vi "Write to Active Buffer.vi"(8 "error in (no error)":errorcluster, 10 "Data":string, 11 "Terminal in":refnum<class "Terminal.lvclass">) -> (0 "error out":errorcluster, 3 "Terminal out":refnum<class "Terminal.lvclass">)   [LabVIEW 2020, in "Terminal.lvlib" / "Terminal.lvclass"]
uses:
  Terminal.lvclass
  Terminal.lvclass/Terminal.ctl
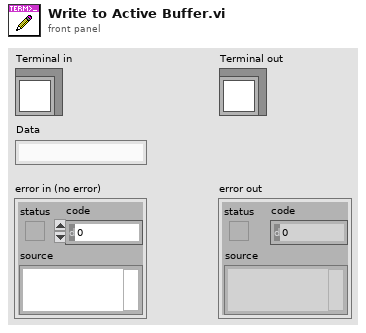
[diagram p1: front panel]
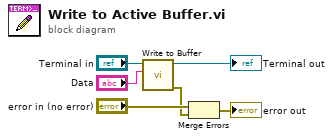
[diagram p0: block diagram]
diagram:
  n1 = call "Write to Buffer.vi"("Data"="Data", "Terminal in"="Terminal in") -> ("error out"=w1:errorcluster, "Terminal out"=→"Terminal out":refnum<class "Terminal.lvclass">)  [unwired: 8 in]
  n2 = Merge Errors("error in (no error)", w1) -> (→"error out":errorcluster)
